vi "Setup.vi"(8 "error in (no error)":errorcluster, 11 "Number of Modules":i32) -> (0 "error out":errorcluster, 1 "Module Routes":refnum<user-event>[](array[refnum]), 3 "Event Refs":refnum<event-registration>[](array[refnum]))   [LabVIEW 2018]
doc: "Setup the application for success!"
uses:
  Message Queue/Message Cluster.ctl
  Message Queue/Message Queue.lvlib
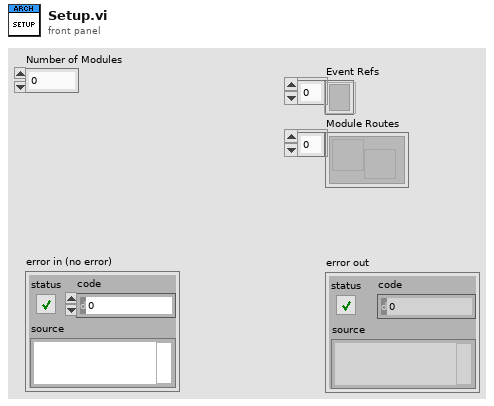
[diagram p1: front panel]
types:
  T1 = typedef "Message Queue.lvlib/Message Cluster.ctl" = cluster{"Message":string, "Message Data":variant}
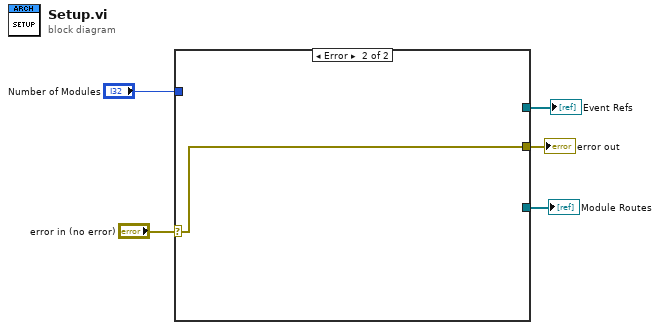
[diagram p0: block diagram]
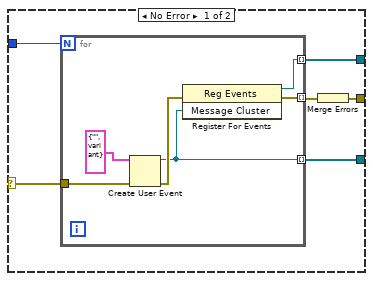
[diagram p2: hidden frame]
diagram:
  n1 = case shown="Error" "error in (no error)" {
    selector: "error in (no error)" -> [w6 w18]
    tunnel: "Number of Modules" -> [w11 _]
    tunnel: [w9 w18] -> w4
    tunnel: [w8 _] -> w3
    tunnel: [w7 _] -> w2
    frame No Error {
      n2 = for {
        N: w11 -> [_]
        tunnel: w6 -> [w17]
        tunnel: [w14] -> w10 mode=indexing
        tunnel: [w13] -> w8 mode=indexing
        tunnel: [w12] -> w7 mode=indexing
        n3 = Create User Event(user event datatype=T1 {"Message"="", "Message Data"=variant} ("Message Cluster"), error in=w17) -> (user event=w12:refnum<user-event>, error out=w15:errorcluster)
        n4 = register-events(error in=w15, w12) -> (reference out=w13:refnum<event-registration>, error out=w14:errorcluster)  [unwired: 1 in]
      }
      n5 = Merge Errors(w10) -> (w9:errorcluster)
    }
    frame Error {
    }
  }
  "error out" <- w4
  "Event Refs" <- w3
  "Module Routes" <- w2
